vi "Download PTC10Log.vi"() -> ()   [LabVIEW 2023]
uses:
  <instrlib>/Stanford PTC10/SRS PTC10.lvlib
panel:
  out "Waveform Graph":waveform(dbl)(graph)
  out "Numeric":i32
  out "Integer output":i32
  out "Output":string
  in  "SRS PTC10 VISA in":refnum<visa-resource-name>="GPIB0::22::INSTR"
  in  "Channel to fetch":string
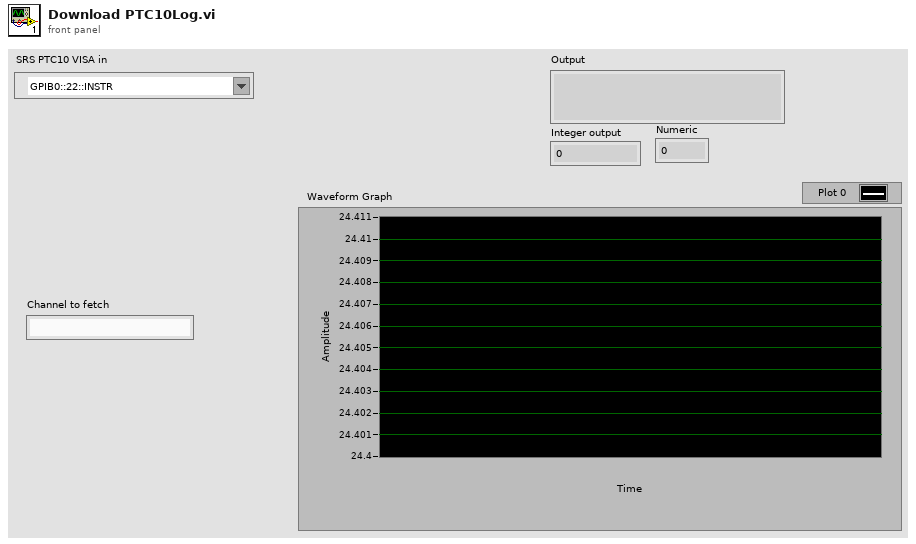
[diagram p1: front panel]
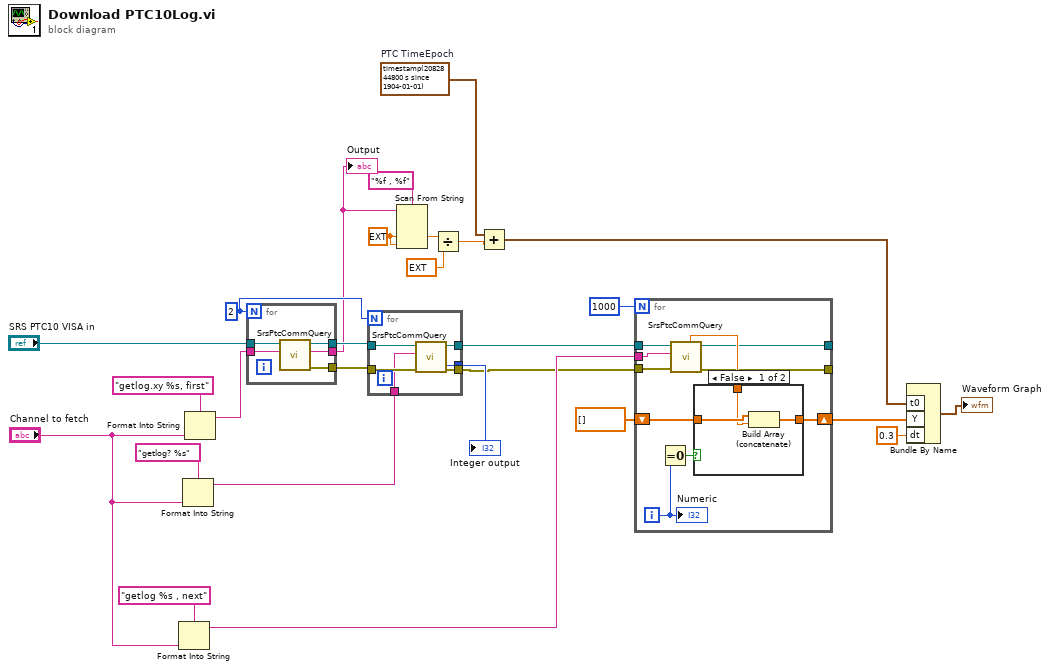
[diagram p0: block diagram]
diagram:
  w6 = timestamp(2082844800 s since 1904-01-01)  # PTC TimeEpoch
  w10 = ext 0.0 ("default value 1")
  w13 = 2
  n1 = Format Into String(format string="getlog %s , next", "Channel to fetch") -> (resulting string=w18:string)  [unwired: 2 in, 1 out]
  n2 = Format Into String(format string="getlog? %s", "Channel to fetch") -> (resulting string=w21:string)  [unwired: 2 in, 1 out]
  n3 = Format Into String(format string="getlog.xy %s, first", "Channel to fetch") -> (resulting string=w25:string)  [unwired: 2 in, 1 out]
  n4 = for {
    N: w13 -> [_]
    tunnel: [w29] -> w23
    tunnel: "SRS PTC10 VISA in" -> [w32]
    tunnel: [w30] -> w24
    tunnel: w25 -> [w31]
    tunnel: [w28] -> w12
    n5 = call <instrlib>:"SrsPtcCommQuery.vi"("Command"=w31, "SRS PTC10 VISA in"=w32) -> ("error out"=w29:errorcluster, "Output"=w28:string, "SRS PTC10 VISA out"=w30:refnum<visa-resource-name>)  [unwired: 4 in, 3 out]
  }
  "Output" <- w12
  n6 = for {
    N: w13 -> [_]
    tunnel: w21 -> [w36]
    tunnel: [w35] -> w20
    tunnel: w23 -> [w37]
    tunnel: [w33] -> w15
    tunnel: w24 -> [w38]
    tunnel: [w34] -> w16
    n7 = call <instrlib>:"SrsPtcCommQuery.vi"("error in"=w37, "Command"=w36, "SRS PTC10 VISA in"=w38) -> ("error out"=w33:errorcluster, "SRS PTC10 VISA out"=w34:refnum<visa-resource-name>, "Integer output"=w35:i32)  [unwired: 3 in, 3 out]
  }
  "Integer output" <- w20
  n8 = Scan From String(format string="%f , %f", input string=w12, default 1=w10, default 2=w10) -> (output 1=w9:ext)  [unwired: 3 in, 3 out]
  n9 = Divide(x=w9, y=ext 1000.0 ("x")) -> (x/y=w7:ext)
  n10 = Add(x=w6, y=w7) -> (x+y=w5:timestamp)
  n11 = for {
    N: 1000 -> [_]
    tunnel: w16 -> [w48]
    tunnel: w18 -> [w47]
    tunnel: w15 -> [w46]
    shift-right: [w44] -> w4
    shift-left: dbl[] [] -> [w45]
    tunnel: [w42] -> _
    tunnel: [w41] -> _
    i -> [w39]
    n12 = Equal To 0?(x=w39) -> (x = 0?=w40:bool)
    n13 = call <instrlib>:"SrsPtcCommQuery.vi"("error in"=w46, "Command"=w47, "SRS PTC10 VISA in"=w48) -> ("error out"=w42:errorcluster, "SRS PTC10 VISA out"=w41:refnum<visa-resource-name>, "Float output"=w43:dbl)  [unwired: 3 in, 3 out]
    n14 = case shown="False" w40 {
      tunnel: w45 -> [w51 w52]
      tunnel: [w50 w52] -> w44
      tunnel: w43 -> [w49 _]
      frame False {
        n15 = Build Array (concatenate)(w51, w49) -> (w50:dbl[])
      }
      frame True {
      }
    }
    "Numeric" <- w39
  }
  n16 = Bundle By Name("t0"=w5, "Y"=w4, "dt"=0.3) -> (→"Waveform Graph":waveform(dbl))  [unwired: 1 in]
